vi "Curtin1_NewTest.vi"(9 "Template name":string, 11 "Settings":T2={"Name of test"="", "Date"=timestamp(0 s since 1904-01-01), "Location"="", "Default Template"="", "Soundcard"="", "resolution"=32, "Sampling rate"=48000, "Ch1 Gain "=25.0, "Ch2 Gain"=10.0, "Sample time (s)"=0.3, "Pre-trigger (s)"=0.01, "Hammer Threshold"=10.0, "Positions"=12, "Taps/Position"=5, "Set Names"="", "Freq resolution"=10.0, "Hammer cutoff"=0.0, "Mic cutoff"=0.0, "Double bounce "=0.0, "Hammer Cal"=10.0, "dB Offset"=0.0, "Accel Cal"=10.0, "Vibrometer Cal"=0.0, "Mic Cal"=0.0, "Output"=2, "Voltage Cal"=0.01, "Vibrometer Port"="ASRL27::INSTR", "Range"=4, "High Pass"=2, "Bandwidth"=4, "X Range"=[{"Minimum"=200.0, "Maximum"=10000.0, "Increment"=10.0, "Minor Increment"=100.0, "Start"=200.0}, {"Minimum"=0.0, "Maximum"=0.05, "Increment"=0.025, "Minor Increment"=0.0025, "Start"=0.0}, {"Minimum"=0.0, "Maximum"=0.3, "Increment"=0.1, "Minor Increment"=0.01, "Start"=0.0}, {"Minimum"=200.0, "Maximum"=10000.0, "Increment"=10.0, "Minor Increment"=100.0, "Start"=1000.0}], "Y Range"=[{"Minimum"=-25.0, "Maximum"=0.0, "Increment"=5.0, "Minor Increment"=1.0, "Start"=-25.0}, {"Minimum"=-0.01, "Maximum"=0.1, "Increment"=0.02, "Minor Increment"=0.005, "Start"=0.0}, {"Minimum"=-0.1, "Maximum"=0.1, "Increment"=0.05, "Minor Increment"=0.01, "Start"=-0.1}, {"Minimum"=-35.0, "Maximum"=5.0, "Increment"=2.0, "Minor Increment"=0.5, "Start"=-34.0}], "dB Spread"=0.0, "Trigger"=0, "Ch_1"=25, "Ch_2"=25, "flip?"=FALSE, "60Hz"=FALSE, "Time Offset"=0.0, "Piezo Cal"=0.0, "Default Notes"="", "Tom"=FALSE} {"Ch_2" min=1 step=1; "Ch_1" min=1 max=100 step=1; "Trigger" items=["Hammer (force)", "Self-tap", "Spacebar"]; "Bandwidth" items=["1 kHz"=1, "5 kHz"=5, "10 kHz"=10, "25 kHz"=25, "50 kHz"=50, "100 kHz"=100]; "High Pass" items=["Off", "13 Hz", "104 Hz"]; "Range" items=["10 mm/s"=1, "20 mm/s"=2, "50 mm/s"=5, "100 mm/s"=10, "200 mm/s"=20, "500 mm/s"=50, "1 m/s"=100, "2 m/s"=200]; "Output" items=["Accelerometer", "Speed (from acceleration)", "Microphone", "Vibrometer"]; "Voltage Cal" format="%#_13g"; "Ch2 Gain" format="%#_13g"; "Ch1 Gain" format="%#_13g"; "Double bounce" min=0.0; "Mic cutoff" min=0.0 format="%#_4g"; "Hammer cutoff" min=0.0 format="%#_4g"; "Freq resolution" min=0.0; "Pre-trigger (s)" format="%#_13g"; "Date" format="%<%H:%M\n%d/%m/%y>T"; "resolution" items=["16 bit"=16, "24 bit"=24, "32 bit"=32]; "Sampling rate" items=["22050 samp/s"=22050, "44100 samp/s"=44100, "48000 samp/s"=48000]}) -> (2 "Success":bool, 3 "Settings Out":T1={"Name of test"="", "Date"=timestamp(0 s since 1904-01-01), "Location"="", "Template"="", "Soundcard"="", "resolution"=32, "Sampling rate"=48000, "Ch1 Gain "=25.0, "Ch2 Gain"=10.0, "Sample time (s)"=0.3, "Pre-trigger (s)"=0.01, "Hammer Threshold"=10.0, "Positions"=12, "Taps/Position"=5, "Set Names"="", "Freq resolution"=10.0, "Hammer cutoff"=0.0, "Mic cutoff"=0.0, "Double bounce "=0.0, "Hammer Cal"=10.0, "dB Offset"=0.0, "Accel Cal"=10.0, "Vibrometer Cal"=0.0, "Mic Cal"=0.0, "Output"=2, "Voltage Cal"=0.01, "Vibrometer Port"="ASRL27::INSTR", "Range"=4, "High Pass"=2, "Bandwidth"=4, "X Range"=[], "Y Range"=[], "dB Spread"=0.0, "Trigger"=0, "Ch_1"=25, "Ch_2"=25, "flip?"=FALSE, "60Hz"=FALSE, "Time offset"=0.0, "Piezo Cal"=1.0, "Default Notes"="", "Tom"=FALSE} {"Ch_2" min=1 step=1; "Ch_1" min=1 max=100 step=1; "Trigger" items=["Hammer (force)", "Self-tap", "Spacebar"]; "Bandwidth" items=["1 kHz"=1, "5 kHz"=5, "10 kHz"=10, "25 kHz"=25, "50 kHz"=50, "100 kHz"=100]; "High Pass" items=["Off", "13 Hz", "104 Hz"]; "Range" items=["10 mm/s"=1, "20 mm/s"=2, "50 mm/s"=5, "100 mm/s"=10, "200 mm/s"=20, "500 mm/s"=50, "1 m/s"=100, "2 m/s"=200]; "Output" items=["Accelerometer", "Speed (from acceleration)", "Microphone", "Vibrometer", "Piezo"]; "Voltage Cal" format="%#_13g"; "Ch2 Gain" format="%#_13g"; "Ch1 Gain" format="%#_13g"; "Double bounce" min=0.0; "Mic cutoff" min=0.0 format="%#_4g"; "Hammer cutoff" min=0.0 format="%#_4g"; "Freq resolution" min=0.0; "Pre-trigger (s)" format="%#_13g"; "Date" format="%<%H:%M\n%d/%m/%y>T"; "resolution" items=["16 bit"=16, "24 bit"=24, "32 bit"=32]; "Sampling rate" items=["22050 samp/s"=22050, "44100 samp/s"=44100, "48000 samp/s"=48000]})   [LabVIEW 2022 SP3]
uses:
  <vilib>/Utility/miscctls.llb/LVSelectionTypeDef.ctl
  Mic/Mic_Global.vi
  PreferencesControl.ctl
panel:
  out "Photos":picture[](array[picture])
  in  "Photo add":bool
  in  "Calib":u16(ring) items=["Use template calibration", "Default", "ModalShop"]
  in  "View":bool
  in  "Update Template":bool
  out "Comparison info":string
  out "String":string="Updating Vibrometer..."
  out "start":T1={"Name of test"="", "Date"=timestamp(0 s since 1904-01-01), "Location"="", "Template"="", "Soundcard"="", "resolution"=0, "Sampling rate"=0, "Ch1 Gain "=25.0, "Ch2 Gain"=10.0, "Sample time (s)"=0.0, "Pre-trigger (s)"=0.0, "Hammer Threshold"=0.0, "Positions"=0, "Taps/Position"=0, "Set Names"="", "Freq resolution"=0.0, "Hammer cutoff"=0.0, "Mic cutoff"=0.0, "Double bounce "=0.0, "Hammer Cal"=0.0, "dB Offset"=0.0, "Accel Cal"=0.0, "Vibrometer Cal"=0.0, "Mic Cal"=0.0, "Output"=0, "Voltage Cal"=1.0, "Vibrometer Port"="ASRL27::INSTR", "Range"=4, "High Pass"=2, "Bandwidth"=4, "X Range"=[], "Y Range"=[], "dB Spread"=0.0, "Trigger"=0, "Ch_1"=25, "Ch_2"=25, "flip?"=FALSE, "60Hz"=FALSE, "Time offset"=0.0, "Piezo Cal"=1.0, "Default Notes"="", "Tom"=FALSE} {"Ch_2" min=1 step=1; "Ch_1" min=1 max=100 step=1; "Trigger" items=["Hammer (force)", "Self-tap", "Spacebar"]; "Bandwidth" items=["1 kHz"=1, "5 kHz"=5, "10 kHz"=10, "25 kHz"=25, "50 kHz"=50, "100 kHz"=100]; "High Pass" items=["Off", "13 Hz", "104 Hz"]; "Range" items=["10 mm/s"=1, "20 mm/s"=2, "50 mm/s"=5, "100 mm/s"=10, "200 mm/s"=20, "500 mm/s"=50, "1 m/s"=100, "2 m/s"=200]; "Output" items=["Accelerometer", "Speed (from acceleration)", "Microphone", "Vibrometer", "Piezo"]; "Voltage Cal" format="%#_13g"; "Ch2 Gain" format="%#_13g"; "Ch1 Gain" format="%#_13g"; "Double bounce" min=0.0; "Mic cutoff" min=0.0 format="%#_4g"; "Hammer cutoff" min=0.0 format="%#_4g"; "Freq resolution" min=0.0; "Pre-trigger (s)" format="%#_13g"; "Date" format="%<%H:%M\n%d/%m/%y>T"; "resolution" items=["16 bit"=16, "24 bit"=24, "32 bit"=32]; "Sampling rate" items=["22050 samp/s"=22050, "44100 samp/s"=44100, "48000 samp/s"=48000]}
  in  "DAQ":bool
  out "current":string
  out "Hammer Spectrum":cluster{dbl, "df":dbl, "FFT {X}":dbl[]}[](graph)=[{0.0, "df"=1.0, "FFT {X}"=array[24000 elements]}, {0.0, "df"=40000.0, "FFT {X}"=[-20.0, -20.0]}]
  out "Hammer Data":cluster{dbl, "dt":dbl, "Y":dbl[]}[](graph)=[{0.0, "dt"=2.0833333333333333e-05, "Y"=array[14400 elements]}, {0.0, "dt"=0.0, "Y"=[]}]
  out "Microphone Data":cluster{dbl, "dt":dbl, "Y":dbl[]}[](graph)=[{0.0, "dt"=2.0833333333333333e-05, "Y"=array[14400 elements]}, {0.0, "dt"=0.0, "Y"=[]}]
  out "Average FRF":cluster{dbl, "df":dbl, dbl[]}[](graph)=[{0.0, "df"=1.0, array[24000 elements]}, {0.0, "df"=1.0, array[24000 elements]}]
  out "Vib Cover":bool
  in  "Vibrometer 2":bool
  in  "Vibrometer":bool
  in  "Save as a Template":bool
  in  "Import Template":bool
  in  "Test":bool
  in  "device:":u16(ring) items=["BuerginBase Microphone", "485B39 200083408035100798118210422", "MacBook Pro Microphone", "Microsoft Teams Audio"]
  in  "OK Button":bool
  in  "Cancel Button":bool
  in  "Instrument Notes":string
  in  "Tag List":bool
  in  "Instrument Name":string(combo)
  in  "Instrument Keywords":string
  out "File name":string
  in  "Test Name":string
  # "New Test"
  # "Adjust default scale ranges"
  # "Adjust default scale ranges"
  # "Hz"
  # "dB"
  # "dB"
  # "sec"
  # "sec"
  # "mV/Pa"
  # "mV/m/s2"
  # "mV/mm/s"
  # "V/N"
  # "sec"
  # "sec"
  # "mV/N"
  # "%"
  # "%"
  # "sec"
  # "mV/Pa"
  # "mV/m/s2"
  # "mV/mm/s"
  # "V/N"
  # "sec"
  # "sec"
  # "mV/N"
  # "Hz"
  # "%"
  # "dB"
  # "%"
  # "dB"
  # "sec"
  # "sec"
  # "sec"
  # "Hz"
  # "dB"
  # "dB"
  # "sec"
  # "sec"
  # "mV/Pa"
  # "mV/m/s2"
  # "mV/mm/s"
  # "V/N"
  # "sec"
  # "sec"
  # "mV/N"
  # "%"
  # "%"
  # "sec"
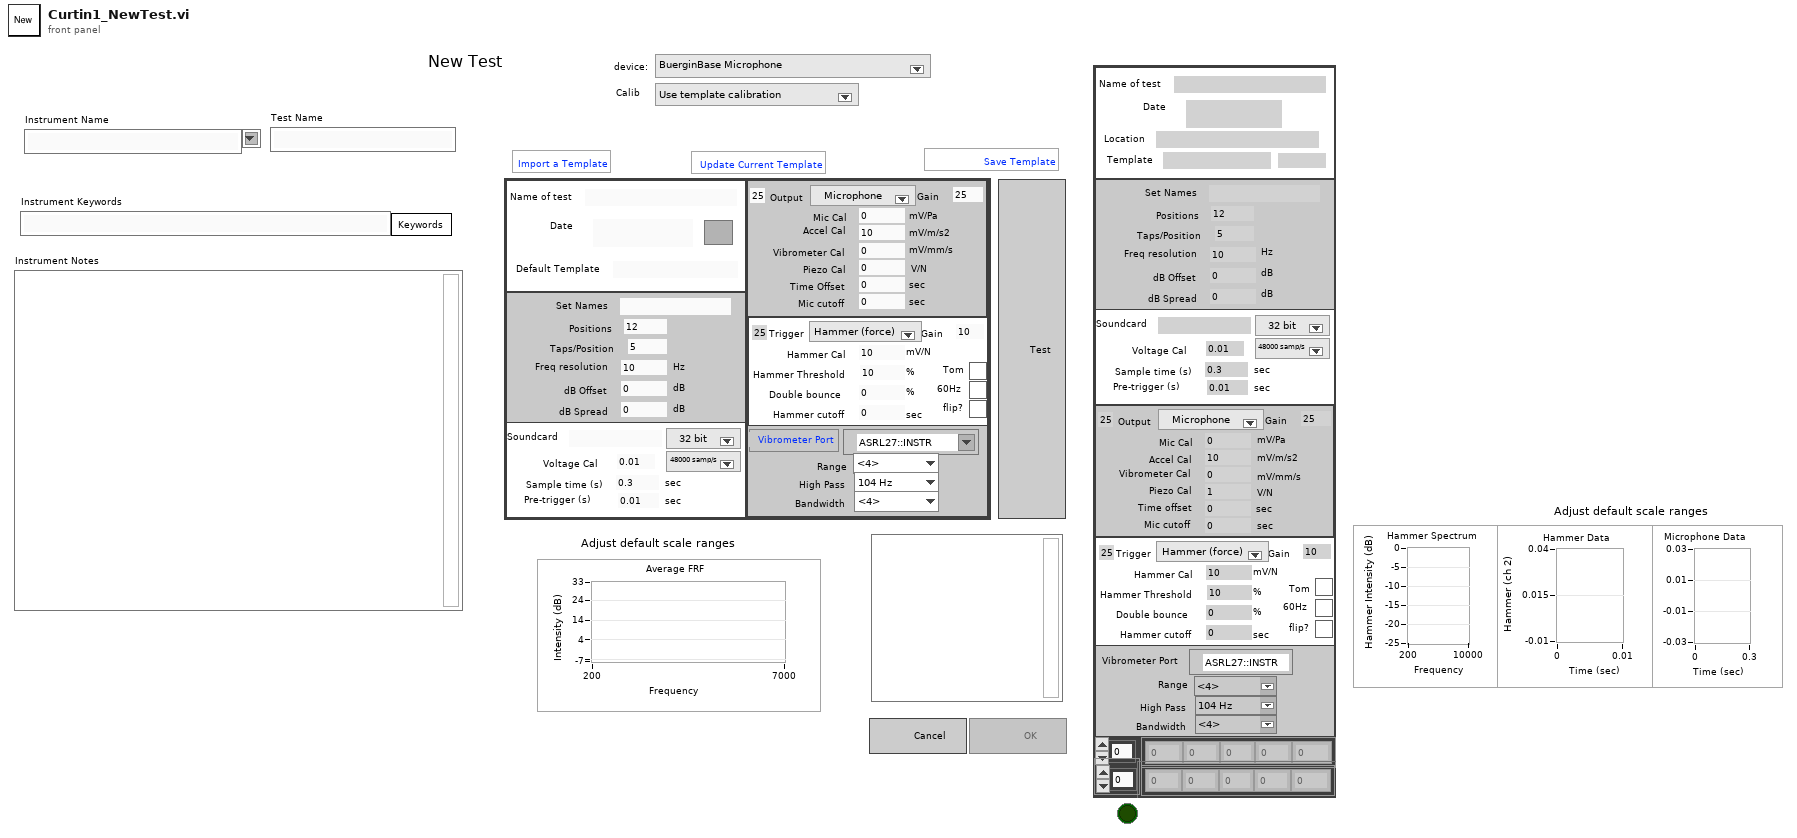
[diagram p1: front panel]
types:
  T1 = typedef "PreferencesControl.ctl" = cluster{"Name of test":string, "Date":timestamp, "Location":string, "Template":string, "Soundcard":string, "resolution":u16, "Sampling rate":u16, "Ch1 Gain ":dbl, "Ch2 Gain":dbl, "Sample time (s)":dbl, "Pre-trigger (s)":dbl, "Hammer Threshold":dbl, "Positions":i16, "Taps/Position":i16, "Set Names":string, "Freq resolution":dbl, "Hammer cutoff":dbl, "Mic cutoff":dbl, "Double bounce ":dbl, "Hammer Cal":dbl, "dB Offset":dbl, "Accel Cal":dbl, "Vibrometer Cal":dbl, "Mic Cal":dbl, "Output":u16, "Voltage Cal":dbl, "Vibrometer Port":refnum<visa-resource-name>, "Range":u16, "High Pass":u16, "Bandwidth":u16, "X Range":cluster{"Minimum":dbl, "Maximum":dbl, "Increment":dbl, "Minor Increment":dbl, "Start":dbl}[], "Y Range":cluster{"Minimum":dbl, "Maximum":dbl, "Increment":dbl, "Minor Increment":dbl, "Start":dbl}[], "dB Spread":dbl, "Trigger":u16, "Ch_1":u8, "Ch_2":u8, "flip?":bool, "60Hz":bool, "Time offset":dbl, "Piezo Cal":dbl, "Default Notes":string, "Tom":bool}
  T2 = cluster{"Name of test":string, "Date":timestamp, "Location":string, "Default Template":string, "Soundcard":string, "resolution":u16, "Sampling rate":u16, "Ch1 Gain ":dbl, "Ch2 Gain":dbl, "Sample time (s)":dbl, "Pre-trigger (s)":dbl, "Hammer Threshold":dbl, "Positions":i16, "Taps/Position":i16, "Set Names":string, "Freq resolution":dbl, "Hammer cutoff":dbl, "Mic cutoff":dbl, "Double bounce ":dbl, "Hammer Cal":dbl, "dB Offset":dbl, "Accel Cal":dbl, "Vibrometer Cal":dbl, "Mic Cal":dbl, "Output":u16, "Voltage Cal":dbl, "Vibrometer Port":refnum<visa-resource-name>, "Range":u16, "High Pass":u16, "Bandwidth":u16, "X Range":cluster{"Minimum":dbl, "Maximum":dbl, "Increment":dbl, "Minor Increment":dbl, "Start":dbl}[], "Y Range":cluster{"Minimum":dbl, "Maximum":dbl, "Increment":dbl, "Minor Increment":dbl, "Start":dbl}[], "dB Spread":dbl, "Trigger":u16, "Ch_1":u8, "Ch_2":u8, "flip?":bool, "60Hz":bool, "Time Offset":dbl, "Piezo Cal":dbl, "Default Notes":string, "Tom":bool}
  T3 = enum8{"Enabled", "Disabled", "Disabled and Grayed Out"}
  T4 = typedef "LVSelectionTypeDef.ctl" = cluster{"Selection Start":u32, "Selection End":u32}
  T5 = typedef "LVRangeTypeDef.ctl" = cluster{"Minimum":dbl, "Maximum":dbl, "Increment":dbl, "Minor Increment":dbl, "Start":dbl}
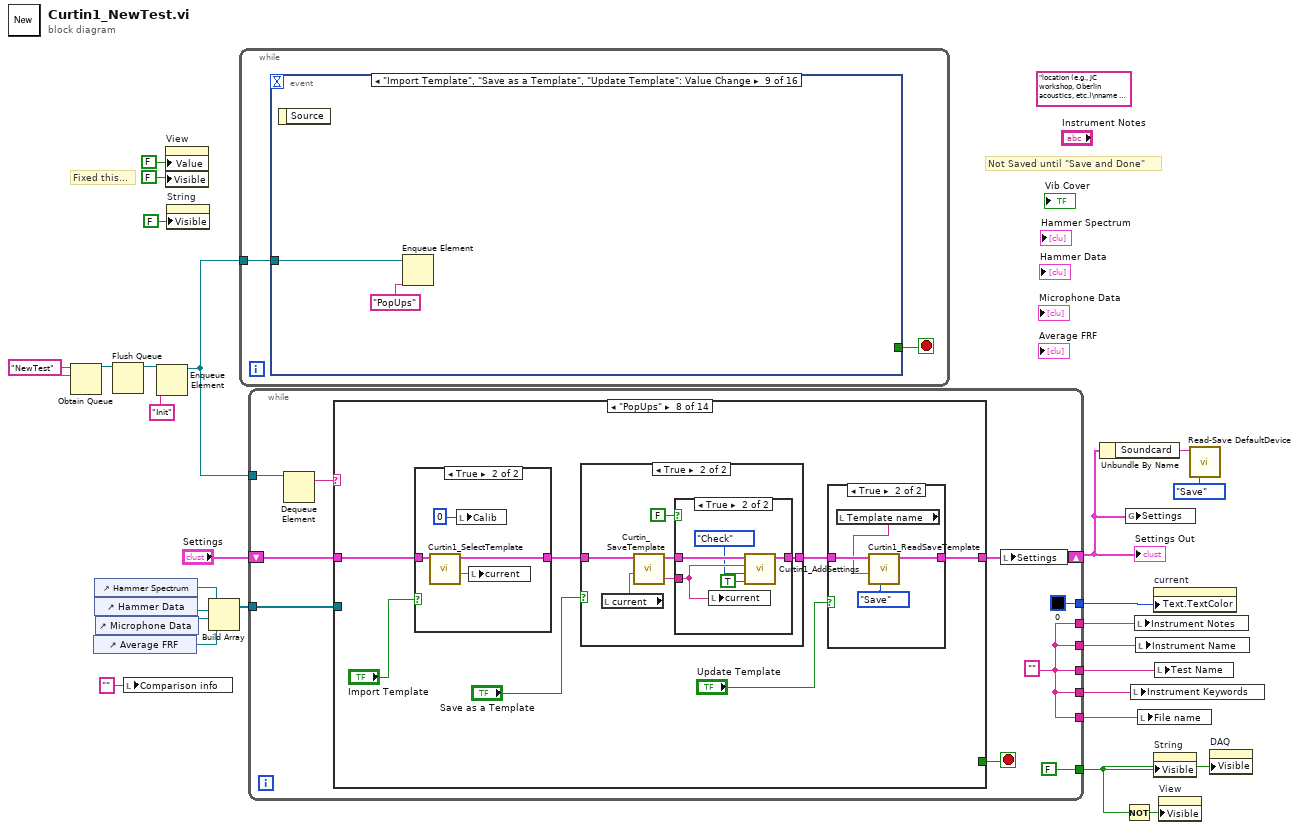
[diagram p0: block diagram]
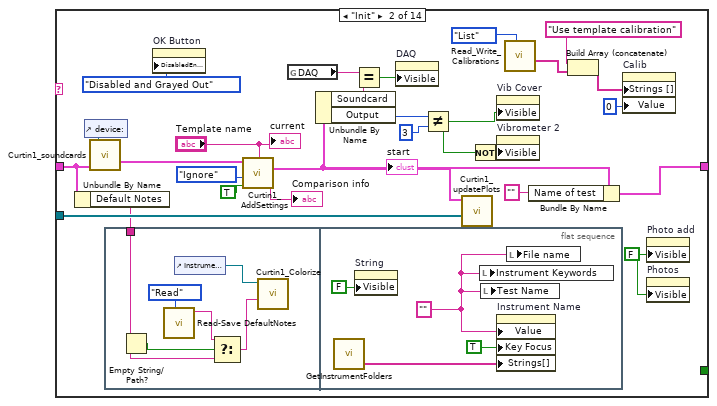
[diagram p3: hidden frame]
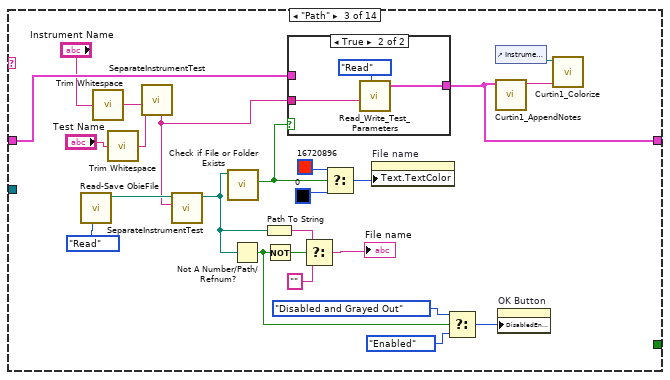
[diagram p4: hidden frame]
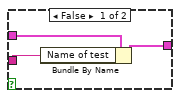
[diagram p5: hidden frame]
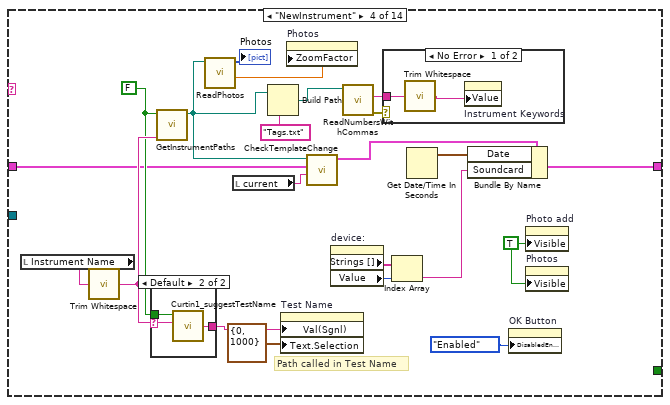
[diagram p6: hidden frame]
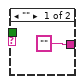
[diagram p8: hidden frame]
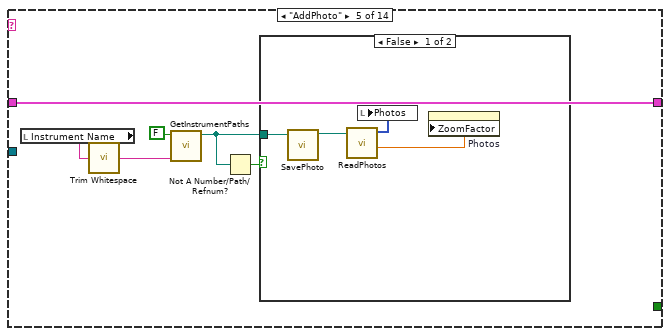
[diagram p9: hidden frame]
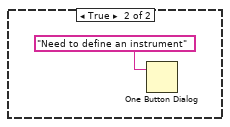
[diagram p10: hidden frame]
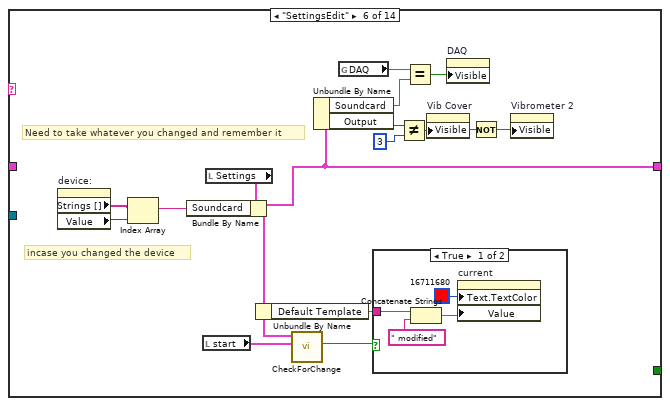
[diagram p11: hidden frame]
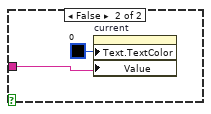
[diagram p12: hidden frame]
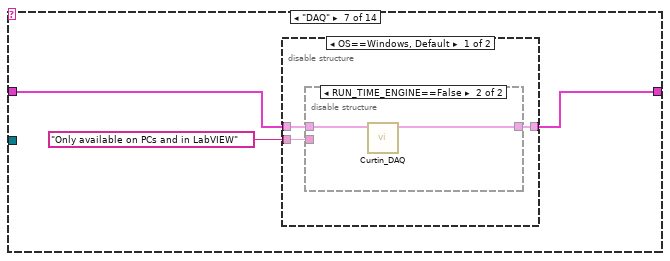
[diagram p13: hidden frame]
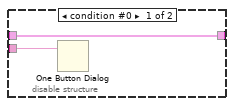
[diagram p14: hidden frame]
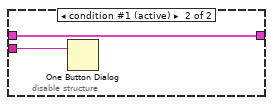
[diagram p15: hidden frame]
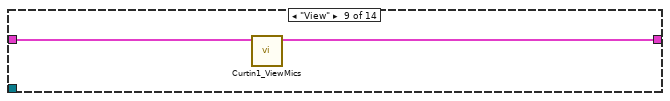
[diagram p20: hidden frame]
diagram:
  (unwired) "location (e.g., JC workshop, Oberlin acoustics, etc.)\nname of experiment (if applicable) \nnames of researchers\n\nInstrument Information:\ninstrument (e.g., violin, viola, cello, guitar, mandolin, etc.) \nmodel (e.g., Titian Strad, Guadagnini, personal, etc.) \nmaker name\nmaker ID (e.g., serial number)\nyear built (4 digits)\ncountry of origin \nsession (e.g. Oberlin 2017, VSA 2008) \nmaking school (e.g. Old Italian) \n\nMeasurement Information:\ntype (Radiation, admittance, modal analysis, taptones, etc.) \nprotocol (HV24, etc.)\n" ("Notes")
  w26 = "NewTest" ("name (unnamed)")
  # "Fixed this..."
  # "Not Saved until \"Save and Done\""
  n1 = Obtain Queue(name (unnamed)=w26, element data type=w26) -> (queue out=w4:refnum<queue>)  [unwired: 3 in, 2 out]
  n2 = control-ref of="Average FRF"() -> (w14:refnum<vi>)
  n3 = control-ref of="Hammer Spectrum"() -> (w17:refnum<vi>)
  n4 = control-ref of="Hammer Data"() -> (w16:refnum<vi>)
  n5 = control-ref of="Microphone Data"() -> (w15:refnum<vi>)
  n6 = Flush Queue(queue=w4) -> (queue out=w3:refnum<queue>)  [unwired: 1 in, 2 out]
  n7 = local write "Comparison info"("" ("Comparison info")) -> ()
  n8 = Enqueue Element(queue=w3, element="Init") -> (queue out=w24:refnum<queue>)  [unwired: 2 in, 2 out]
  n9 = property on="View" class="Bool (strict)"("Value"=FALSE ("View"), "Visible"=FALSE) -> ()  [unwired: 2 in, 2 out]
  n10 = property on="String" class="Str"("Visible"=FALSE) -> ()  [unwired: 2 in, 2 out]
  n11 = Build Array(w17, w16, w15, w14) -> (w13:refnum<vi>[])
  n12 = while {
    tunnel: w24 -> [w27]
    stop <- w28 stop-if-true
    n13 = event shown="[8] \"Import Template\", \"Save as a Template\", \"Update Template\": Value Change" {
      selector: _ -> [_ _ _ _ _ _ _ _ _ _ _ _ _ _ _ _]
      dyn-events: _ -> [_ _ _ _ _ _ _ _ _ _ _ _ _ _ _ _]
      timeout: _ -> [_ _ _ _ _ _ _ _ _ _ _ _ _ _ _ _]
      tunnel: [_ _ _ _ _ _ _ _ _ _ _ _ TRUE w57 _ _] -> w28
      tunnel: w27 -> [_ w29 w31 _ w34 w36 w38 w40 w42 w44 w46 w48 w54 w59 _ w76]
      event Timeout {
        n14 = event-data() -> ()  [unwired: 1 in, 3 out]
      }
      event "Test Name": Value Change {
        n15 = event-data() -> ()  [unwired: 1 in, 1 out]
        n16 = Enqueue Element(queue=w29, element="Path") -> ()  [unwired: 2 in, 3 out]
      }
      event "Settings": Value Change {
        n17 = event-data() -> ()  [unwired: 1 in, 1 out]
        n18 = Enqueue Element(queue=w31, element="SettingsEdit") -> ()  [unwired: 2 in, 3 out]
      }
      event "View": Value Change {
        w33 = FALSE ("Visible")
        n19 = event-data() -> ()  [unwired: 1 in, 1 out]
        n20 = property on="View" class="Bool (strict)"("Value"=w33, "Visible"=w33) -> ()  [unwired: 2 in, 2 out]
      }
      event "Instrument Name": Value Change {
        n21 = event-data() -> ()  [unwired: 1 in, 1 out]
        n22 = Enqueue Element(queue=w34, element="NewInstrument") -> ()  [unwired: 2 in, 3 out]
      }
      event "device:": Value Change {
        n23 = event-data() -> ()  [unwired: 1 in, 6 out]
        n24 = Enqueue Element(queue=w36, element="SettingsEdit") -> ()  [unwired: 2 in, 3 out]
      }
      event "DAQ": Value Change {
        n25 = event-data() -> ()  [unwired: 1 in, 6 out]
        n26 = Enqueue Element(queue=w38, element="DAQ") -> ()  [unwired: 2 in, 3 out]
      }
      event "Calib": Value Change {
        n27 = event-data() -> ()  [unwired: 1 in, 1 out]
        n28 = Enqueue Element(queue=w40, element="Calib") -> ()  [unwired: 2 in, 3 out]
      }
      event "Import Template", "Save as a Template", "Update Template": Value Change {
        n29 = event-data() -> ()  [unwired: 1 in, 1 out]
        n30 = Enqueue Element(queue=w42, element="PopUps") -> ()  [unwired: 2 in, 3 out]
      }
      event "Test": Value Change {
        n31 = event-data() -> ()  [unwired: 1 in, 6 out]
        n32 = Enqueue Element(queue=w44, element="View") -> ()  [unwired: 2 in, 3 out]
      }
      event "Average FRF", "Microphone Data", "Hammer Data", "Hammer Spectrum": Scale Range Change {
        n33 = event-data() -> ()  [unwired: 1 in, 8 out]
        n34 = Enqueue Element(queue=w46, element="Scales") -> ()  [unwired: 2 in, 3 out]
      }
      event "Vibrometer", "Vibrometer 2": Value Change {
        n35 = event-data() -> ()  [unwired: 1 in, 6 out]
        n36 = Enqueue Element(queue=w48, element="Vibrometer") -> ()  [unwired: 2 in, 3 out]
      }
      event "OK Button", "Cancel Button": Value Change {
        n37 = event-data() -> ()  [unwired: 1 in, 6 out]
        n38 = Select(t="Save and Done" ("element"), s="OK Button", f="Done" ("element")) -> (s? t:f=w51:string)
        n39 = Enqueue Element(queue=w54, element=w51) -> ()  [unwired: 2 in, 3 out]
        "Success" <- "OK Button"
      }
      event Panel Close? {
        w57 = TRUE
        n40 = event-data() -> ()  [unwired: 1 in, 4 out]
        n41 = Enqueue Element(queue=w59, element="Done") -> ()  [unwired: 2 in, 3 out]
        n42 = local write "Success"(FALSE ("Success")) -> ()
        n43 = event-data("Discard?"=w57) -> ()  [unwired: 1 in, 1 out]
      }
      event "Tag List", "Instrument Keywords": Value Change {
        n44 = event-data() -> ()  [unwired: 1 in, 1 out]
        n45 = case shown="True" "Tag List" {
          tunnel: ["" ("Tags out") w75] -> w64
          frame False {
          }
          frame True {
            n46 = call "RequestTags.vi"() -> ("Tags out"=w75:string)  [unwired: 11 in]
          }
        }
        n47 = case shown="Default" "Instrument Keywords" {
          tunnel: w64 -> [w65 w66]
          tunnel: "Instrument Keywords" -> [_ w68]
          tunnel: [w65 w67] -> w62
          frame "" {
          }
          frame Default {
            n48 = case shown="Default" w66 {
              selector: w66 -> [_ w70]
              tunnel: w68 -> [w69 w73]
              tunnel: [w69 w72] -> w67
              frame "" {
              }
              frame Default {
                n49 = Concatenate Strings(w73, "," ("string"), w70) -> (w72:string)
              }
            }
          }
        }
        n50 = call "RemoveDuplicateTags.vi"("Tags"=w62) -> ("Tag string"=w60:string)  [unwired: 9 in, 1 out]
        n51 = local write "Instrument Keywords"(w60) -> ()
      }
      event "Photo add": Value Change {
        n52 = event-data() -> ()  [unwired: 1 in, 1 out]
        n53 = Enqueue Element(queue=w76, element="AddPhoto") -> ()  [unwired: 2 in, 3 out]
      }
    }
  }
  n54 = while {
    tunnel: w24 -> [w85]
    shift-right: [w78] -> w6
    shift-left: "Settings" -> [w83]
    tunnel: [w82] -> w23
    tunnel: [w82] -> w22
    tunnel: [w82] -> w21
    tunnel: [w82] -> w20
    tunnel: [w82] -> w19
    tunnel: [FALSE ("Visible")] -> w8
    tunnel: w13 -> [w80]
    tunnel: [u32 0 ("Text.Text Colors:Text Color")] -> w12
    stop <- w84 stop-if-true
    w82 = "" ("Value (Signaling)")
    n55 = Dequeue Element(queue=w85) -> (element=w86:string)  [unwired: 2 in, 3 out]
    n56 = case shown="\"PopUps\"" w86 {
      tunnel: [_ _ _ _ _ _ _ _ _ _ _ _ TRUE TRUE] -> w84
      tunnel: w83 -> [w87 w96 w131 w165 w187 _ w215 w226 w257 w259 w264 w267 w282 w287]
      tunnel: [w87 w112 w128 w170 w187 w198 w214 w228 w256 w258 w263 w266 w282 w284] -> w78
      tunnel: w80 -> [_ w99 _ _ _ _ _ _ _ w260 _ _ _ _]
      frame Default {
      }
      frame "Init" {
        w88 = FALSE ("Visible")
        n57 = Unbundle By Name(w96) -> ("Default Notes"=w95:string)
        n58 = control-ref of="device:"() -> (w113:refnum<vi>)
        n59 = call "Curtin1_soundcards.vi"("Settings In"=w96, "device:"=w113) -> ("Settings Out"=w97:T1)  [unwired: 8 in, 1 out]
        n60 = flat-sequence {
          tunnel: w95 -> [w115]
          frame #0 {
            n61 = Empty String/Path?(string/path=w115) -> (empty?=w114:bool)
            n62 = call "Read-Save DefaultNotes.vi"("Task"=enum16{"Save", "Read"}."Read") -> ("Notes Out"=w117:string)  [unwired: 9 in, 1 out]
            n63 = control-ref of="Instrument Notes"() -> (w118:refnum<vi>)
            n64 = Select(t=w117, s=w114, f=w115) -> (s? t:f=w116:string)
            n65 = call "Curtin1_Colorize.vi"("Instrument Notes"=w116, "Text"=w118) -> ()  [unwired: 10 in]
          }
          frame #1 {
            w121 = "" ("Value (Signaling)")
            n66 = call "GetInstrumentFolders.vi"() -> ("folder names"=w123:string[])  [unwired: 11 in]
            n67 = property on="String" class="Str"("Visible"=FALSE) -> ()  [unwired: 2 in, 2 out]
            n68 = local write "Instrument Keywords"(w121) -> ()
            n69 = local write "Test Name"(w121) -> ()
            n70 = property on="Instrument Name" class="CmbBox"("Value"=w121, "Key Focus"=TRUE, "Strings[]"=w123) -> ()  [unwired: 2 in, 2 out]
            n71 = local write "File name"(w121) -> ()
          }
        }
        n72 = property on="OK Button" class="Bool"("DisabledEnum"=T3."Disabled and Grayed Out" ("Disabled")) -> ()  [unwired: 2 in, 2 out]
        n73 = call "Curtin1_AddSettings.vi"("Date?"=TRUE, "Check?"=enum16{"Ignore", "Check", "Replace"}."Ignore", "Template"="Template name", "Settings in"=w97) -> ("text"=→"Comparison info":string, "Settings Out"=w98:T1)  [unwired: 6 in]
        "start" <- w98
        n74 = global read "Mic_Global.vi" "DAQ"() -> (w105:string)
        n75 = Unbundle By Name(w98) -> ("Soundcard"=w104:string, "Output"=w110:u16)
        n76 = Equal?(x=w105, y=w104) -> (x = y?=w103:bool)
        n77 = property on="DAQ" class="Bool"("Visible"=w103) -> ()  [unwired: 2 in, 2 out]
        n78 = Not Equal?(x=w110, y=u16 3) -> (x != y?=w108:bool)
        n79 = call "Curtin1_updatePlots.vi"("plots"=w99, "Settings"=w98) -> ()  [unwired: 10 in]
        n80 = Not(x=w108) -> (.not. x?=w107:bool)
        n81 = property on="Vib Cover" class="Bool (strict)"("Visible"=w108) -> ()  [unwired: 2 in, 2 out]
        n82 = property on="Vibrometer 2" class="Bool"("Visible"=w107) -> ()  [unwired: 2 in, 2 out]
        n83 = call "Read_Write_Calibrations.vi"("Task"=enum16{"Save", "Read", "List"}."List") -> ("Cal files"=w93:string[])  [unwired: 8 in, 2 out]
        n84 = Bundle By Name(cluster=w98, "Name of test"="") -> (w112:T1)
        n85 = Build Array (concatenate)("Use template calibration", w93) -> (w92:string[])
        n86 = property on="Calib" class="Ring (strict)"("Strings []"=w92, "Value"=0) -> ()  [unwired: 2 in, 2 out]
        n87 = property on="Photo add" class="Bool"("Visible"=w88) -> ()  [unwired: 2 in, 2 out]
        n88 = property on="Photos" class="Arr (strict)"("Visible"=w88) -> ()  [unwired: 2 in, 2 out]
        "current" <- "Template name"
      }
      frame "Path" {
        n89 = call "Read-Save ObieFile.vi"("Task"=enum16{"Save", "Read"}."Read") -> ("DataPath Out"=w134:path)  [unwired: 8 in, 2 out]
        n90 = call <vilib>:"Trim Whitespace.vi"("string"="Instrument Name") -> ("trimmed string"=w127:string)  [unwired: 1 in]
        n91 = call <vilib>:"Trim Whitespace.vi"("string"="Test Name") -> ("trimmed string"=w124:string)  [unwired: 1 in]
        n92 = call "SeparateInstrumentTest.vi"("test in"=w124, "Instrument in"=w127) -> ("Instrument -- test out"=w132:string)  [unwired: 5 in, 4 out]
        n93 = call "SeparateInstrumentTest.vi"("Instrument"=w132, "path in"=w134) -> ("path out"=w133:path)  [unwired: 5 in, 4 out]
        n94 = call <vilib>:"Check if File or Folder Exists.vi"("path"=w133) -> ("file or folder exists?"=w136:bool)  [unwired: 8 in, 2 out]
        n95 = Not A Number/Path/Refnum?(number/path/refnum=w133) -> (NaN/Path/Refnum?=w146:bool)
        n96 = Path To String(path=w133) -> (string=w145:string)
        n97 = Not(x=w146) -> (.not. x?=w144:bool)
        n98 = case shown="True" w136 {
          tunnel: w131 -> [w150 _]
          tunnel: [w149 w151] -> w128
          tunnel: w132 -> [w148 w152]
          frame False {
            n99 = Bundle By Name(cluster=w150, "Name of test"=w148) -> (w149:T1)
          }
          frame True {
            n100 = call "Read_Write_Test_Parameters.vi"("Task"=enum16{"Save", "Read", "Clear"}."Read", "Instrument Name"=w152) -> ("Settings"=w151:T1)  [unwired: 8 in, 1 out]
          }
        }
        n101 = Select(t=w145, s=w144, f="") -> (s? t:f=→"File name":string)
        n102 = Select(t=u32 16720896, s=w136, f=u32 0) -> (s? t:f=w143:u32)
        n103 = property on="File name" class="Str"("Text.TextColor"=w143) -> ()  [unwired: 2 in, 2 out]
        n104 = Select(t=T3."Disabled and Grayed Out" ("Disabled"), s=w146, f=T3."Enabled" ("Disabled")) -> (s? t:f=w147:T3)
        n105 = control-ref of="Instrument Notes"() -> (w130:refnum<vi>)
        n106 = call "Curtin1_AppendNotes.vi"("Settings"=w128) -> ("Instrument Notes"=w129:string)  [unwired: 10 in]
        n107 = property on="OK Button" class="Bool"("DisabledEnum"=w147) -> ()  [unwired: 2 in, 2 out]
        n108 = call "Curtin1_Colorize.vi"("Instrument Notes"=w129, "Text"=w130) -> ()  [unwired: 10 in]
      }
      frame "NewInstrument" {
        w155 = TRUE ("Visible")
        w167 = FALSE ("Build?")
        # "Path called in Test Name"
        n109 = local read "Instrument Name"() -> (w172:string)
        n110 = call <vilib>:"Trim Whitespace.vi"("string"=w172) -> ("trimmed string"=w171:string)  [unwired: 1 in]
        n111 = case shown="Default" w171 {
          selector: w171 -> [_ w181]
          tunnel: ["" w180] -> w175
          tunnel: w167 -> [_ w179]
          frame "" {
          }
          frame Default {
            n112 = call "Curtin1_suggestTestName.vi"("instrument"=w181, "Build?"=w179) -> ("Suggested Test"=w180:string)  [unwired: 9 in]
          }
        }
        n113 = call "GetInstrumentPaths.vi"("Instrument"=w171, "Build?"=w167) -> ("Path To Instrument Folder"=w157:path)  [unwired: 5 in, 4 out]
        n114 = call "ReadPhotos.vi"("Path To Instrument Folder"=w157) -> ("zoom"=w154:dbl, "photos"=→"Photos":picture[])  [unwired: 9 in]
        n115 = local read "current"() -> (w161:string)
        n116 = Build Path(base path=w157, name or relative path="Tags.txt") -> (appended path=w160:path)
        n117 = property on="Test Name" class="Str"("Val(Sgnl)"=w175, "Text.Selection"=T4 {"Selection Start"=0, "Selection End"=1000}) -> ()  [unwired: 2 in, 2 out]
        n118 = property on="Photos" class="Pict"("ZoomFactor"=w154) -> ()  [unwired: 2 in, 2 out]
        n119 = call "CheckTemplateChange.vi"("Template"=w161, "Settings In"=w165, "Path To Instrument Folder"=w157) -> ("Settings  Out"=w162:T1)  [unwired: 7 in, 1 out]
        n120 = property on="device:" class="Ring (strict)"() -> ("Strings []"=w168:string[], "Value"=w169:u16)  [unwired: 2 in, 2 out]
        n121 = call "ReadNumbersWithCommas.vi"("file (use dialog)"=w160) -> ("error out"=w158:errorcluster, "text"=w159:string)  [unwired: 7 in, 2 out]
        n122 = case shown="No Error" w158 {
          tunnel: w159 -> [w177 _]
          frame No Error {
            n123 = call <vilib>:"Trim Whitespace.vi"("string"=w177) -> ("trimmed string"=w176:string)  [unwired: 1 in]
            n124 = property on="Instrument Keywords" class="Str"("Value"=w176) -> ()  [unwired: 2 in, 2 out]
          }
          frame Error {
          }
        }
        n125 = Index Array(array=w168, index=w169) -> (element=w164:string)
        n126 = Get Date/Time In Seconds() -> (seconds since 1Jan1904=w163:timestamp)
        n127 = Bundle By Name(cluster=w162, "Date"=w163, "Soundcard"=w164) -> (w170:T1)
        n128 = property on="OK Button" class="Bool"("DisabledEnum"=T3."Enabled" ("Disabled")) -> ()  [unwired: 2 in, 2 out]
        n129 = property on="Photo add" class="Bool"("Visible"=w155) -> ()  [unwired: 2 in, 2 out]
        n130 = property on="Photos" class="Arr (strict)"("Visible"=w155) -> ()  [unwired: 2 in, 2 out]
      }
      frame "AddPhoto" {
        n131 = local read "Instrument Name"() -> (w186:string)
        n132 = call <vilib>:"Trim Whitespace.vi"("string"=w186) -> ("trimmed string"=w185:string)  [unwired: 1 in]
        n133 = call "GetInstrumentPaths.vi"("Instrument"=w185, "Build?"=FALSE) -> ("Path To Instrument Folder"=w182:path)  [unwired: 5 in, 4 out]
        n134 = Not A Number/Path/Refnum?(number/path/refnum=w182) -> (NaN/Path/Refnum?=w183:bool)
        n135 = case shown="False" w183 {
          tunnel: w182 -> [w191 _]
          frame False {
            n136 = call "SavePhoto.vi"("Instrument path"=w191) -> ("Instrument out"=w188:path)  [unwired: 10 in]
            n137 = call "ReadPhotos.vi"("Path To Instrument Folder"=w188) -> ("zoom"=w190:dbl, "photos"=w189:picture[])  [unwired: 9 in]
            n138 = local write "Photos"(w189) -> ()
            n139 = property on="Photos" class="Pict"("ZoomFactor"=w190) -> ()  [unwired: 2 in, 2 out]
          }
          frame True {
            n140 = One Button Dialog(message="Need to define an instrument") -> ()  [unwired: 1 in, 1 out]
          }
        }
      }
      frame "SettingsEdit" {
        # "incase you changed the device"
        # "Need to take whatever you changed and remember it"
        n141 = property on="device:" class="Ring (strict)"() -> ("Strings []"=w206:string[], "Value"=w207:u16)  [unwired: 2 in, 2 out]
        n142 = Index Array(array=w206, index=w207) -> (element=w204:string)
        n143 = local read "start"() -> (w193:T1)
        n144 = local read "Settings"() -> (w205:T2)
        n145 = Bundle By Name(cluster=w205, "Soundcard"=w204) -> (w198:T2)
        n146 = Unbundle By Name(w198) -> ("Default Template"=w199:string)
        n147 = call "CheckForChange.vi"("Original Settings"=w193, "Current Settings"=w198) -> ("change?"=w197:bool)  [unwired: 8 in, 1 out]
        n148 = Unbundle By Name(w198) -> ("Soundcard"=w194:string, "Output"=w203:u16)
        n149 = global read "Mic_Global.vi" "DAQ"() -> (w196:string)
        n150 = case shown="True" w197 {
          tunnel: w199 -> [w208 w212]
          frame True {
            n151 = Concatenate Strings(w208, " modified" ("string")) -> (w209:string)
            n152 = property on="current" class="Str"("Text.TextColor"=u32 16711680 ("Text.Text Colors:Text Color"), "Value"=w209) -> ()  [unwired: 2 in, 2 out]
          }
          frame False {
            n153 = property on="current" class="Str"("Text.TextColor"=u32 0 ("Text.Text Colors:Text Color"), "Value"=w212) -> ()  [unwired: 2 in, 2 out]
          }
        }
        n154 = Not Equal?(x=w203, y=u16 3) -> (x != y?=w202:bool)
        n155 = Equal?(x=w196, y=w194) -> (x = y?=w195:bool)
        n156 = property on="Vib Cover" class="Bool (strict)"("Visible"=w202) -> ()  [unwired: 2 in, 2 out]
        n157 = property on="DAQ" class="Bool"("Visible"=w195) -> ()  [unwired: 2 in, 2 out]
        n158 = Not(x=w202) -> (.not. x?=w200:bool)
        n159 = property on="Vibrometer 2" class="Bool"("Visible"=w200) -> ()  [unwired: 2 in, 2 out]
      }
      frame "DAQ" {
        n160 = disable-structure shown="OS==Windows, Default" {
          disable-tunnel: "Only available on PCs and in LabVIEW" ("message") -> [w219 w225]
          disable-tunnel: w215 -> [w218 w224]
          disable-tunnel: [w217 w224] -> w214
          frame condition #0 {
            n161 = disable-structure shown="RUN_TIME_ENGINE==False" {
              disable-tunnel: w219 -> [w221 _]
              disable-tunnel: w218 -> [w220 w223]
              disable-tunnel: [w220 w222] -> w217
              frame condition #0 {
                n162 = One Button Dialog(message=w221) -> ()  [unwired: 1 in, 1 out]
              }
              frame condition #1 (active) {
                n163 = call "Curtin_DAQ.vi"("Settings"=w223) -> ("Settings out"=w222:T1)  [unwired: 10 in]
              }
            }
          }
          frame condition #1 (active) {
            n164 = One Button Dialog(message=w225) -> ()  [unwired: 1 in, 1 out]
          }
        }
      }
      frame "PopUps" {
        n165 = case shown="True" "Import Template" {
          tunnel: w226 -> [w251 w255]
          tunnel: [w251 w253] -> w230
          frame False {
          }
          frame True {
            n166 = call "Curtin1_SelectTemplate.vi"("Settings in"=w255) -> ("New Template"=w254:string, "Settings out"=w253:T1)  [unwired: 9 in]
            n167 = local write "Calib"(0) -> ()
            n168 = local write "current"(w254) -> ()
          }
        }
        n169 = case shown="True" "Save as a Template" {
          tunnel: [w238 w241] -> w229
          tunnel: w230 -> [w238 w244]
          frame False {
          }
          frame True {
            n170 = local read "current"() -> (w240:string)
            n171 = call "Curtin_SaveTemplate.vi"("Template Name"=w240, "Settings in"=w244) -> ("New Template"=w242:string, "Settings out"=w243:T1)  [unwired: 7 in, 1 out]
            n172 = case shown="True" FALSE {
              tunnel: w243 -> [w245 w250]
              tunnel: w242 -> [_ w248]
              tunnel: [w245 w249] -> w241
              frame False {
              }
              frame True {
                n173 = local write "current"(w248) -> ()
                n174 = call "Curtin1_AddSettings.vi"("Date?"=TRUE, "Check?"=enum16{"Ignore", "Check", "Replace"}."Check", "Template"=w248, "Settings in"=w250) -> ("Settings Out"=w249:T1)  [unwired: 6 in, 1 out]
              }
            }
          }
        }
        n175 = case shown="True" "Update Template" {
          tunnel: w229 -> [w233 w236]
          tunnel: [w233 w235] -> w228
          frame False {
          }
          frame True {
            n176 = local read "Template name"() -> (w234:string)
            n177 = call "Curtin1_ReadSaveTemplate.vi"("Task"=enum16{"Save", "Read", "List"}."Save", "Template"=w234, "Settings"=w236) -> ("Settings out"=w235:T1)  [unwired: 5 in, 3 out]
          }
        }
      }
      frame "View" {
        n178 = call "Curtin1_ViewMics.vi"("Settings"=w257) -> ("Settings Out"=w256:T1)  [unwired: 10 in]
      }
      frame "Scales" {
        n179 = call "GetPlotRanges.vi"("plots"=w260) -> ("Yscales"=w262:T5[], "Xscales"=w261:T5[])  [unwired: 9 in]
        n180 = Bundle By Name(cluster=w259, "X Range"=w261, "Y Range"=w262) -> (w258:T1)
      }
      frame "Vibrometer" {
        n181 = call "PolyTec_Control_Panel.vi"("Settings in"=w264) -> ("Settings Out"=w263:T1)  [unwired: 8 in, 2 out]
      }
      frame "Calib" {
        n182 = case shown="0" "Calib" {
          tunnel: "Calib" -> [_ w278]
          tunnel: w267 -> [w271 w275]
          tunnel: [w269 w274] -> w266
          frame 0 {
            n183 = local read "Template name"() -> (w270:string)
            n184 = call "Curtin1_AddSettings.vi"("Date?"=TRUE, "Check?"=enum16{"Ignore", "Check", "Replace"}."Ignore", "Template"=w270, "Settings in"=w271) -> ("Settings Out"=w269:T1)  [unwired: 6 in, 1 out]
          }
          frame Default {
            n185 = property on="Calib" class="Ring (strict)"() -> ("Strings []"=w277:string[])  [unwired: 2 in, 2 out]
            n186 = Index Array(array=w277, index=w278) -> (element=w276:string)
            n187 = call "Read_Write_Calibrations.vi"("Silent?"=TRUE, "Task"=enum16{"Save", "Read", "List"}."Read", "Calibration name"=w276, "Settings in"=w275) -> ("file"=w273:string, "Settings out"=w274:T1)  [unwired: 5 in, 1 out]
            n188 = local write "Comparison info"(w273) -> ()
          }
        }
        n189 = disable-structure shown="Disabled" {
          frame Disabled {
            n190 = call "Curtin1_SelectCalib.vi"("Save?"=FALSE) -> ()  [unwired: 10 in, 1 out]
          }
          frame Enabled {
          }
        }
      }
      frame "Done" {
      }
      frame "Save and Done" {
        n191 = local read "Instrument Keywords"() -> (w288:string)
        n192 = Get Date/Time In Seconds() -> (seconds since 1Jan1904=w291:timestamp)
        n193 = local read "Instrument Notes"() -> (w289:string)
        n194 = Bundle By Name(cluster=w287, "Date"=w291) -> (w285:T1)
        n195 = call "Read_Write_Test_Parameters.vi"("Task"=enum16{"Save", "Read", "Clear"}."Save", "Settings"=w285) -> ()  [unwired: 8 in, 2 out]
        n196 = call "Curtin1_SaveTagsFile.vi"("Tags"=w288, "Settings in"=w285) -> ()  [unwired: 10 in]
        n197 = call "Curtin1_SaveNotesFile.vi"("Notes"=w289, "Settings in"=w285) -> ()  [unwired: 10 in]
        n198 = call "Curtin1_SaveLastSettingsFile.vi"("Settings in"=w285) -> ()  [unwired: 11 in]
        n199 = Unbundle By Name(w285) -> ("Output"=w286:u16)
        n200 = case shown="3" w286 {
          tunnel: w285 -> [w293 w297]
          tunnel: [w293 w295] -> w284
          frame 0, Default {
          }
          frame 3 {
            n201 = call "OverallControl.vi"("Settings"=w297) -> ("Success?"=w298:bool, "VISA Refnum out"=w296:refnum<visa-resource-name>)  [unwired: 9 in]
            n202 = property on="String" class="Str"("Visible"=TRUE) -> ()  [unwired: 2 in, 2 out]
            n203 = case shown="True" w298 {
              tunnel: w297 -> [w299 w303]
              tunnel: w296 -> [_ w302]
              tunnel: [w299 w301] -> w295
              frame False {
                n204 = One Button Dialog(message="Vibrometer not responding") -> ()  [unwired: 1 in, 1 out]
              }
              frame True {
                n205 = Bundle By Name(cluster=w303, "Vibrometer Port"=w302) -> (w301:T1)
              }
            }
          }
        }
      }
    }
    n206 = local write "Settings"(w78) -> ()
  }
  "Settings Out" <- w6
  n207 = Unbundle By Name(w6) -> ("Soundcard"=w5:string)
  n208 = Not(x=w8) -> (.not. x?=w10:bool)
  n209 = global write "Mic_Global.vi" "Settings"(w6) -> ()
  n210 = local write "Instrument Keywords"(w20) -> ()
  n211 = local write "Instrument Notes"(w23) -> ()
  n212 = local write "Instrument Name"(w22) -> ()
  n213 = local write "File name"(w19) -> ()
  n214 = property on="current" class="Str"("Text.TextColor"=w12) -> ()  [unwired: 2 in, 2 out]
  n215 = property on="String" class="Str"("Visible"=w8) -> ()  [unwired: 2 in, 2 out]
  n216 = local write "Test Name"(w21) -> ()
  n217 = property on="View" class="Bool (strict)"("Visible"=w10) -> ()  [unwired: 2 in, 2 out]
  n218 = call "Read-Save DefaultDevice.vi"("Task"=enum16{"Save", "Read"}."Save", "Soundcard"=w5) -> ()  [unwired: 8 in, 2 out]
  n219 = property on="DAQ" class="Bool"("Visible"=w8) -> ()  [unwired: 2 in, 2 out]
